vi "Get N Objects.vi"(8 "error in":errorcluster, 10 "instrument objects":refnum<class "Abstract_Instrument.lvclass">[](array[class]), 11 "pin_names":string[](array[string])) -> (0 "error out":errorcluster, 3 "function objects":refnum<class "Measure_Voltage.lvclass">[](array[class]))   [LabVIEW 2021, in "Measure_Voltage.lvclass"]
uses:
  Measure_Voltage.lvclass
  Instruments/Abstract_Instrument/Abstract_Instrument.lvclass
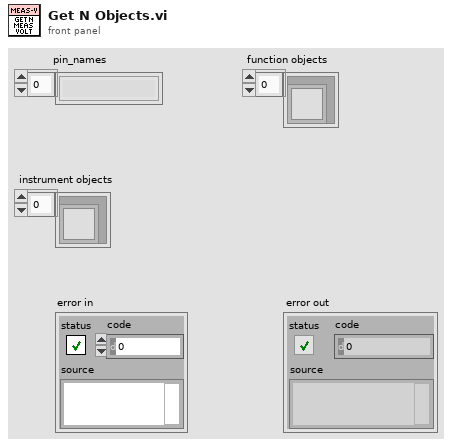
[diagram p1: front panel]
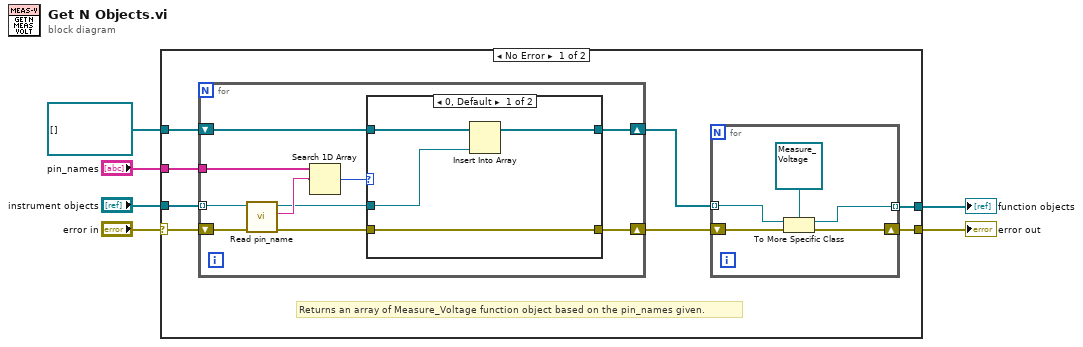
[diagram p0: block diagram]
diagram:
  n1 = case shown="No Error" "error in" {
    selector: "error in" -> [w11 w36]
    tunnel: [w14 w36] -> w6
    tunnel: [w13 _] -> w5
    tunnel: "instrument objects" -> [w10 _]
    tunnel: "pin_names" -> [w9 _]
    tunnel: refnum<class "Abstract_Instrument.lvclass">[] [] ("instrument objects") -> [w8 _]
    frame No Error {
      # "Returns an array of Measure_Voltage function object based on the pin_names given."
      n2 = for {
        shift-right: [w19] -> w12
        shift-left: w11 -> [w24]
        tunnel: w10 -> [w23] mode=indexing
        tunnel: w9 -> [w22]
        shift-right: [w15] -> w7
        shift-left: w8 -> [w16]
        n3 = call-dynamic "Read pin_name.vi"("error in (no error)"=w24, "Abstract_Instrument in"=w23) -> ("error out"=w20:errorcluster, "pin_name"=w18:string, "Abstract_Instrument out"=w17:refnum<class "Abstract_Instrument.lvclass">)  [unwired: 7 in]
        n4 = Search 1D Array(1D array=w22, element=w18) -> (index of element=w21:i32)  [unwired: 1 in]
        n5 = case shown="0, Default" w21 {
          tunnel: w20 -> [w28 w29]
          tunnel: [w28 w29] -> w19
          tunnel: w17 -> [w27 _]
          tunnel: w16 -> [w26 w30]
          tunnel: [w25 w30] -> w15
          frame 0, Default {
            n6 = Insert Into Array(array=w26, new element=w27) -> (w25:refnum<class "Abstract_Instrument.lvclass">[])  [unwired: 1 in]
          }
          frame -1 {
          }
        }
      }
      n7 = for {
        shift-right: [w34] -> w14
        shift-left: w12 -> [w32]
        tunnel: [w33] -> w13 mode=indexing
        tunnel: w7 -> [w31] mode=indexing
        n8 = To More Specific Class(target class=refnum<class "Measure_Voltage.lvclass"> refnum ("Measure_Voltage.lvclass"), reference=w31, error in=w32) -> (specific class reference=w33:refnum<class "Measure_Voltage.lvclass">, error out=w34:errorcluster)
      }
    }
    frame Error {
    }
  }
  "error out" <- w6
  "function objects" <- w5
